vi "setUp.vi"(8 "error in (no error)":errorcluster, 11 "reference in":refnum<class "SystemTestCase.lvclass">=refnum) -> (0 "error out":errorcluster, 3 "reference out":refnum<class "SystemTestCase.lvclass">)   [LabVIEW 2017, in "SystemTestCase.lvclass"]
doc: "setUp runs prior to the test method during test execution. Use this method to initialize any object data required by your tests."
uses:
  SystemTestCase.lvclass
  <vilib>/addons/_JKI Toolkits/VI Tester/TestCase.llb/TestCase.lvclass
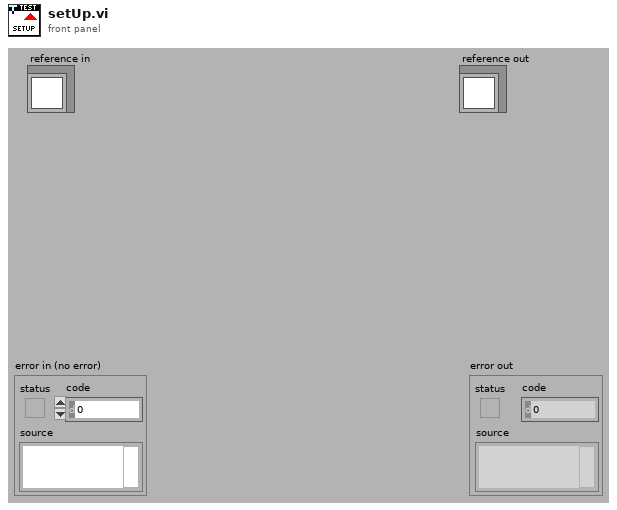
[diagram p1: front panel]
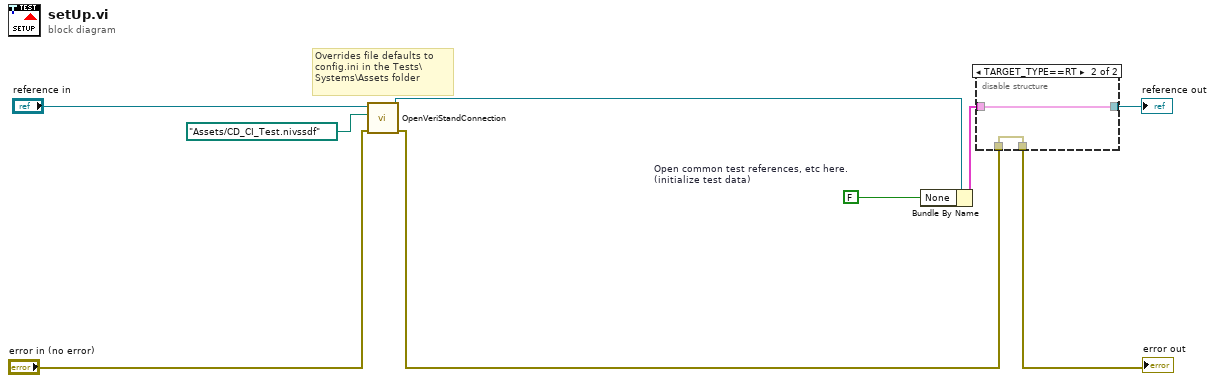
[diagram p0: block diagram]
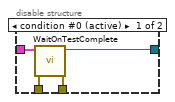
[diagram p2: hidden frame]
diagram:
  w6 = FALSE  # Open common test references, etc here. (initialize test data)
  # "Overrides file defaults to config.ini in the Tests\\Systems\\Assets folder"
  n1 = call-dynamic "OpenVeriStandConnection.vi"("error in (no error)"="error in (no error)", "System Definition File"=path "Assets/CD_CI_Test.nivssdf", "VeriStand Test Case in"="reference in") -> ("error out"=w3:errorcluster, "VeriStand Test Case out"=w4:refnum<class "SystemTestCase.lvclass">)  [unwired: 6 in, 1 out]
  n2 = Bundle By Name(cluster=w4, "None"=w6) -> (w7:cluster{})
  n3 = disable-structure shown="TARGET_TYPE==RT" {
    disable-tunnel: w3 -> [w13 w14]
    disable-tunnel: [w12 w14] -> w9
    disable-tunnel: [w11 w15] -> w8
    disable-tunnel: w7 -> [w10 w15]
    frame condition #0 (active) {
      n4 = call <vilib>:"WaitOnTestComplete.vi"("error in (no error)"=w13, "TestCase in"=w10) -> ("error out"=w12:errorcluster, "TestCase out"=w11:refnum<class "TestCase.lvclass">)  [unwired: 8 in]
    }
    frame condition #1 {
    }
  }
  "error out" <- w9
  "reference out" <- w8
